vi "Test Not Broadcasting Log When Inactive.vi"(8 "error in (no error)":errorcluster, 11 "Test Case In":refnum<class "Debugger Test.lvclass">) -> (0 "error out":errorcluster, 3 "Test Case Out":refnum<class "Debugger Test.lvclass">)   [LabVIEW 2020, in "Debugger Test.lvclass"]
uses:
  Debugger Test.lvclass
  Debugger Test.lvclass/Debugger Test.ctl
  source/Process/Debug Process.lvclass
  source/Debugger/Debugger.lvclass
  C:/Users/anton/Documents/GitHub/triarc-debugger/source/Process/Debug Process.lvclass
  C:/Users/anton/Documents/GitHub/triarc-debugger/source/Debugger/Debugger.lvclass
  C:/Users/anton/Documents/GitHub/triarc-debugger/source/Debug Data Event/Debug Data Listener.lvclass
  source/Debug Data/Debug Data.lvclass
  source/Debug Data/Raw Debug Data.ctl
  ca9a5842-5027-4a08-ae2f-52c95865b329.vi
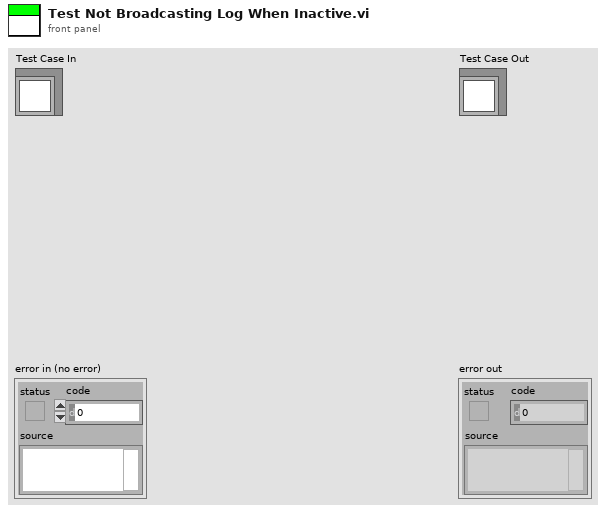
[diagram p1: front panel]
types:
  T1 = typedef "Debug Data.lvclass/Raw Debug Data.ctl" = cluster{"Action":string, "Call Chain":string, "Process":string, "Message":string, "Message Data":variant, "Time":u32}
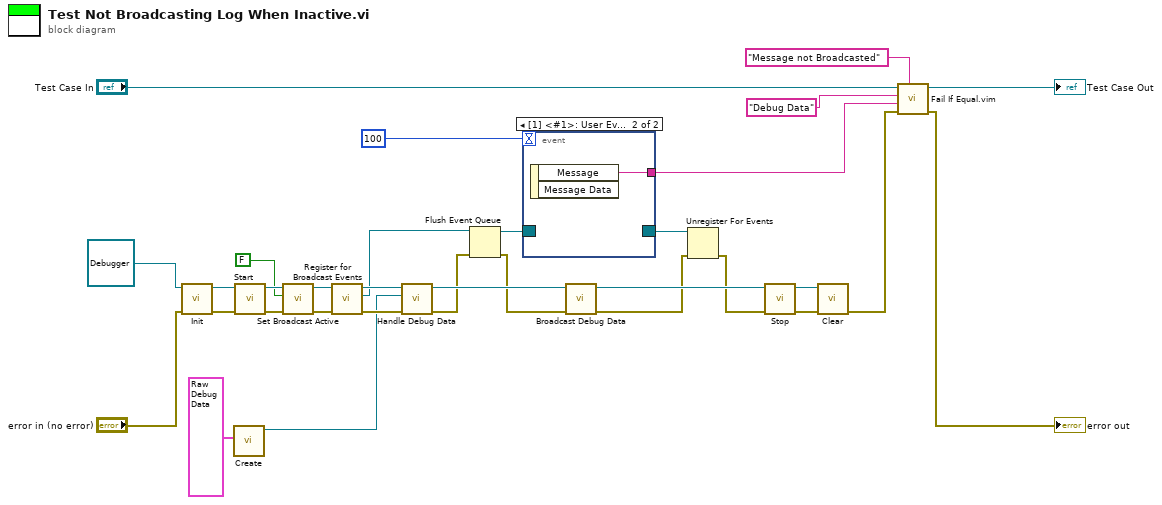
[diagram p0: block diagram]
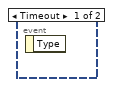
[diagram p2: hidden frame]
diagram:
  n1 = call-dynamic "Init.vi"("error in (no error)"="error in (no error)", "Process In"=refnum<class "Debugger.lvclass"> refnum ("Debug Data Event In 2")) -> ("error out"=w28:errorcluster, "Process Out"=w29:refnum<class "Debugger.lvclass">)  [unwired: 8 in]
  n2 = call "Create.vi"("Debug Data Cluster"=T1 {"Action"="", "Call Chain"="", "Process"="Test", "Message"="", "Message Data"=variant, "Time"=0}) -> ("Debug Data out"=w16:refnum<class "Debug Data.lvclass">)  [unwired: 9 in, 1 out]
  n3 = call "Start.vi"("error in (no error)"=w28, "Process In"=w29) -> ("error out"=w27:errorcluster, "Process Out"=w3:refnum<class "Debugger.lvclass">)  [unwired: 7 in, 1 out]
  n4 = call "Set Broadcast Active.vi"("error in (no error)"=w27, "Active?"=FALSE, "Debugger In"=w3) -> ("error out"=w4:errorcluster, "Debugger Out"=w2:refnum<class "Debugger.lvclass">)  [unwired: 7 in]
  n5 = call "Register for Broadcast Events.vi"("error in (no error)"=w4, "Process In"=w2) -> ("error out"=w26:errorcluster, "Event Registration Refnum Out"=w8:refnum<event-registration>, "Process Out"=w20:refnum<class "Debugger.lvclass">)  [unwired: 7 in]
  n6 = call-dynamic "Handle Debug Data.vi"("error in (no error)"=w26, "Debug Data.lvclass"=w16, "Debug Data Event In"=w20) -> ("error out"=w24:errorcluster, "Debug Data Event Out"=w25:refnum<class "Debugger.lvclass">)  [unwired: 7 in]
  n7 = Flush Event Queue(0:w8, 3:w24) -> (8:w7:refnum<event-registration>, 11:w9:errorcluster)  [unwired: 4 in, 1 out]
  n8 = event shown="[1] <#1>: User Event" {
    selector: w7 -> [_ _]
    dyn-events: [_ _] -> w13
    timeout: 100 -> [_ _]
    tunnel: [_ w33] -> w12
    event Timeout {
      n9 = event-data() -> ()  [unwired: 1 in, 1 out]
    }
    event User Event {
      n10 = event-data() -> ("Message"=w33:string)  [unwired: 1 in, 1 out]
    }
  }
  n11 = call "Broadcast Debug Data.vi"("error in (no error)"=w9, "Debugger in"=w25) -> ("error out"=w6:errorcluster, "Debugger out"=w23:refnum<class "Debugger.lvclass">)  [unwired: 8 in]
  n12 = Unregister For Events(event registration refnum=w13, error in=w6) -> (error out=w5:errorcluster)
  n13 = call "Stop.vi"("error in (no error)"=w5, "Process In"=w23) -> ("error out"=w21:errorcluster, "Process Out"=w22:refnum<class "Debugger.lvclass">)  [unwired: 7 in, 1 out]
  n14 = call-dynamic "Clear.vi"("error in (no error)"=w21, "Process In"=w22) -> ("error out"=w17:errorcluster)  [unwired: 9 in]
  n15 = call "Fail If Equal.vim"("Description"="Message not Broadcasted", "error in (no error)"=w17, "Actual"=w12, "Expected"="Debug Data", "LUnit Test Case In"="Test Case In") -> ("error out"=→"error out":errorcluster, "LUnit Test Case Out"=→"Test Case Out":refnum<class "Debugger Test.lvclass">)  [unwired: 5 in]
